vi "UT_EField_DAQ_AnalogIO.contents.vi"   [LabVIEW 2014, in "UT_EField_DAQ_AnalogIO.lvlib"]
uses:
  UT_EField_DAQ_AnalogIO.lvlib
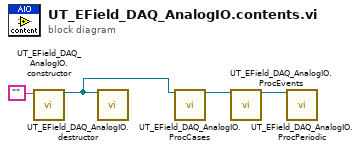
[diagram p0: block diagram]
diagram:
  n1 = call "UT_EField_DAQ_AnalogIO.constructor.vi"("name"="") -> ("i ref out"=w2:refnum<vi>)  [unwired: 16 in, 2 out]
  n2 = call "UT_EField_DAQ_AnalogIO.destructor.vi"("i ref in"=w2) -> ()  [unwired: 18 in, 1 out]
  n3 = call "UT_EField_DAQ_AnalogIO.ProcCases.vi"("i ref in"=w2) -> ("i ref out"=w4:refnum<vi>)  [unwired: 16 in, 2 out]
  n4 = call "UT_EField_DAQ_AnalogIO.ProcEvents.vi"("i ref in"=w4) -> ("i ref out"=w3:refnum<vi>)  [unwired: 17 in, 1 out]
  n5 = call "UT_EField_DAQ_AnalogIO.ProcPeriodic.vi"("i ref in"=w3) -> ()  [unwired: 16 in, 3 out]
